vi "3) Different Data Types.vi"() -> ()   [LabVIEW 2018]
panel:
  out "String 2":string
  in  "String":string
  out "Boolean 2":bool
  in  "Boolean":bool
  in  "Floating Point":dbl
  in  "Integer":dbl
  out "Integer2":dbl
  out "Floating Point2":dbl
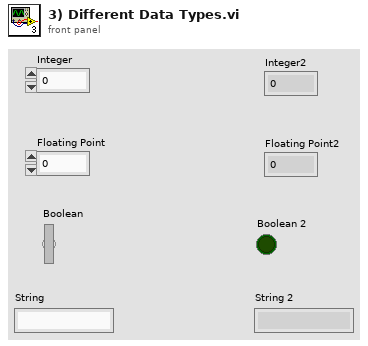
[diagram p1: front panel]
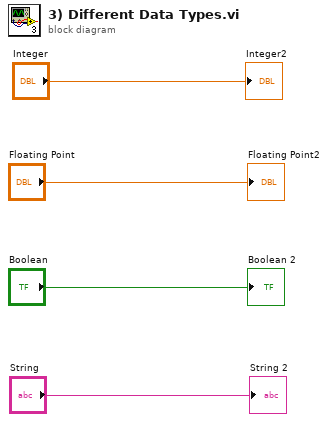
[diagram p0: block diagram]
diagram:
  "Floating Point2" <- "Floating Point"
  "Integer2" <- "Integer"
  "Boolean 2" <- "Boolean"
  "String 2" <- "String"
